vi "Read Arm.vi"(8 "error in (no error)":errorcluster, 11 "Fault-Injection_Boolean in":refnum<class "Fault-Injection_U8.lvclass">) -> (0 "error out":errorcluster, 2 "Armed?":bool, 3 "Fault-Injection_Boolean out":refnum<class "Fault-Injection_U8.lvclass">)   [LabVIEW 2021, in "Fault-Injection_U8.lvclass"]
uses:
  Fault-Injection_U8.lvclass
  Fault-Injection_U8.lvclass/Fault-Injection_U8.ctl
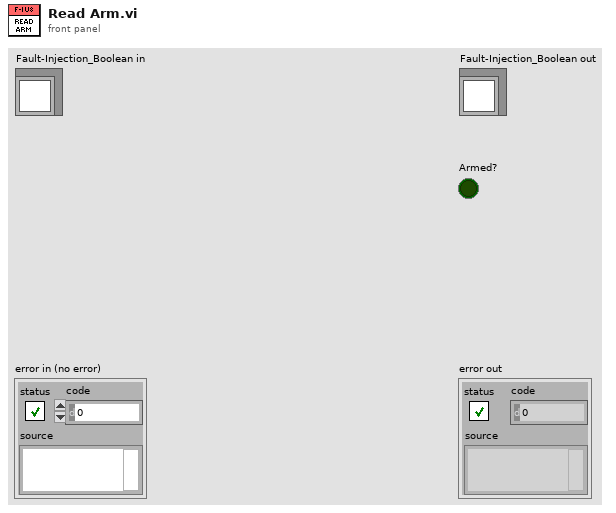
[diagram p1: front panel]
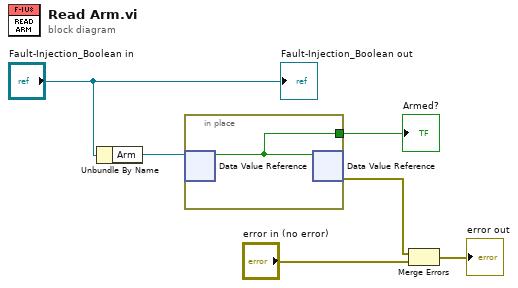
[diagram p0: block diagram]
diagram:
  n1 = Unbundle By Name("Fault-Injection_Boolean in") -> ("Arm"=w5:refnum<data-value>)
  n2 = in-place {
    in-place-border: [w7] -> w4
    n3 = in-place-dvr #1(w5) -> (w7:bool)  [unwired: 1 out]
    n4 = in-place-dvr #1(w7) -> (w2:errorcluster)  [unwired: 1 out]
  }
  "Armed?" <- w4
  n5 = Merge Errors(w2, "error in (no error)") -> (→"error out":errorcluster)
  "Fault-Injection_Boolean out" <- "Fault-Injection_Boolean in"
